vi "SECoP_dataGetEnumeration.vi"(7 "Position":u32, 8 "error in (no error)":errorcluster, 9 "Index":u32, 10 "SECoP_dataPtr in":T1 {"ptr64" format="%.0x"; "ptr32" format="%.0x"}, 11 "DLL path (in)":T2) -> (0 "error out":errorcluster, 1 "enumeration_name":string, 2 "Enumval":i64, 3 "DLL path (out)":T2)   [LabVIEW 2023, in "SECoP.lvlib"]
doc: "Call <b>\"SECoP_dataGetEnumeration.vi\"</b> to access the name and value of an enumeration of a complex data type.\n\n<b>DLL path</b> input and output of cluster from \"SECoP-Initialize.vi\"\n<b>SECoP_dataPtr</b> data to access\n<b>Position</b> points to a virtual flattened entry of the data type; for a simple enumeration use 0\n<b>Index</b> index of the enumeration (starting with 0 to \"SECoP_dataGetEnumerationCount.vi\" - 1)\n<b>EnumVal</b> integer value of requested enumeration\n<b>enumeration_name</b> name of the requested enumeration"
uses:
  SECoP.lvlib
  SECoP-libraries.ctl
  SECoP-data.ctl
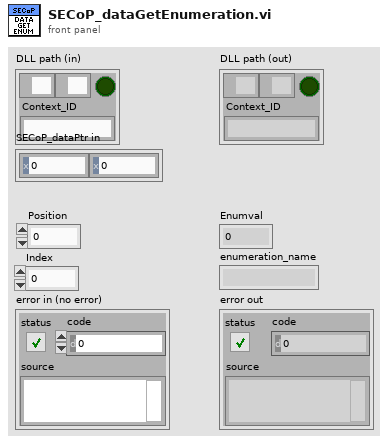
[diagram p1: front panel]
types:
  T1 = typedef "SECoP.lvlib/SECoP-data.ctl" = cluster{"ptr32":u32, "ptr64":u64}
  T2 = typedef "SECoP.lvlib/SECoP-libraries.ctl" = cluster{"serverDLL":path, "variantDLL":path, "cleanup_mode":bool, "Context_ID":string}
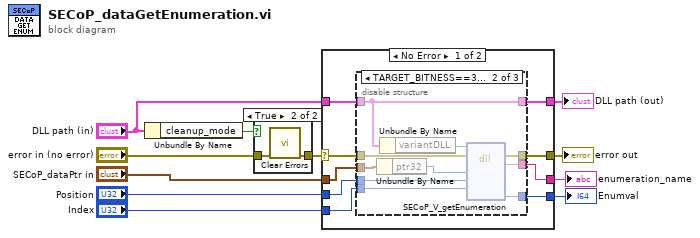
[diagram p0: block diagram]
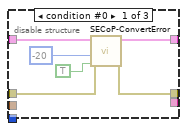
[diagram p3: hidden frame]
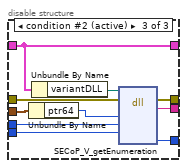
[diagram p4: hidden frame]
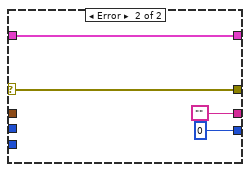
[diagram p5: hidden frame]
diagram:
  n1 = Unbundle By Name("DLL path (in)") -> ("cleanup_mode"=w8:bool)
  n2 = case shown="True" w8 {
    tunnel: "error in (no error)" -> [w12 w14]
    tunnel: [w12 w13] -> w6
    frame False {
    }
    frame True {
      n3 = call <vilib>:"Clear Errors.vi"("error in (no error)"=w14) -> ("error out"=w13:errorcluster)  [unwired: 5 in, 1 out]
    }
  }
  n4 = case shown="No Error" w6 {
    selector: w6 -> [w23 w52]
    tunnel: "DLL path (in)" -> [w22 w53]
    tunnel: [w17 w53] -> w10
    tunnel: [w18 w52] -> w9
    tunnel: "Position" -> [w21 _]
    tunnel: "Index" -> [w20 _]
    tunnel: [w19 i64 0 ("Value")] -> w3
    tunnel: [w16 ""] -> w2
    tunnel: "SECoP_dataPtr in" -> [w15 _]
    frame No Error {
      n5 = disable-structure shown="TARGET_BITNESS==32" {
        disable-tunnel: w23 -> [w27 w39 w49]
        disable-tunnel: w22 -> [w29 w31 w41]
        disable-tunnel: w21 -> [_ w38 w48]
        disable-tunnel: w20 -> [_ w37 w47]
        disable-tunnel: [_ w36 w46] -> w19
        disable-tunnel: [w24 w35 w45] -> w18
        disable-tunnel: [w28 w31 w41] -> w17
        disable-tunnel: [_ w34 w44] -> w16
        disable-tunnel: w15 -> [_ w33 w43]
        frame condition #0 {
          n6 = call "SECoP-ConvertError.vi"("return is boolean"=TRUE, "return code"=-20, "error in (no error)"=w27, "DLL path (in)"=w29) -> ("error out"=w24:errorcluster, "DLL path (out)"=w28:T2)  [unwired: 6 in]
        }
        frame condition #1 {
          n7 = Unbundle By Name(w33) -> ("ptr32"=w32:u32)
          n8 = Unbundle By Name(w31) -> ("variantDLL"=w30:path)
          n9 = dll-call lib="Z:/Praktische_Aufgaben/SECoP-LabVIEW2015/32bit/SECoP32.dll" fn="SECoP_V_getEnumeration"(path in=w30, error in=w39, "Data"=w32, "Position"=w38, "Index"=w37) -> (error out=w35:errorcluster, "return type"=w34:string, "EnumVal"=w36:i64)  [unwired: 5 in, 1 out]
        }
        frame condition #2 (active) {
          n10 = Unbundle By Name(w43) -> ("ptr64"=w42:u64)
          n11 = Unbundle By Name(w41) -> ("variantDLL"=w40:path)
          n12 = dll-call lib="Z:/Praktische_Aufgaben/SECoP-LabVIEW2015/32bit/SECoP32.dll" fn="SECoP_V_getEnumeration"(path in=w40, error in=w49, "Data"=w42, "Position"=w48, "Index"=w47) -> (error out=w45:errorcluster, "return type"=w44:string, "EnumVal"=w46:i64)  [unwired: 5 in, 1 out]
        }
      }
    }
    frame Error {
    }
  }
  "DLL path (out)" <- w10
  "error out" <- w9
  "Enumval" <- w3
  "enumeration_name" <- w2
